vi "Constants.vi"() -> ()   [LabVIEW 2023]
panel:
  in  "Data Length":dbl=9.0
  in  "Current Command Code":string="Code"
  in  "Target Port":u16=6955
  in  "Local Port":u16=6950
  in  "Traget IP Address":string="localhost"
  in  "Local IP Address":string="localhost"
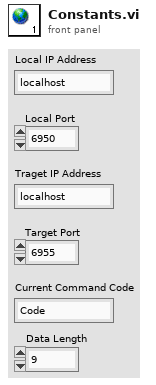
[diagram p1: front panel]
diagram:
